vi "CMN_TrimStringWhitespace.vi"(9 "Both Ends?(T)":bool=TRUE, 10 "string":string) -> (3 "trimmed string":string)   [LabVIEW 2016]
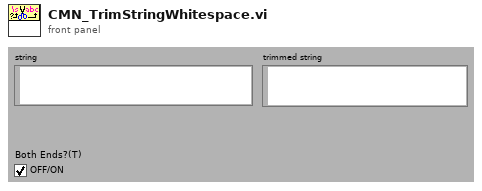
[diagram p1: front panel]
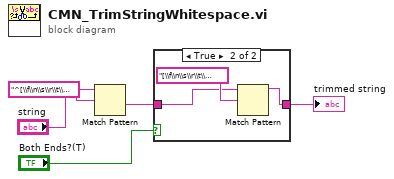
[diagram p0: block diagram]
diagram:
  n1 = Match Pattern(string="string", regular expression="^[\\f\\n\\s\\r\\t\\00]*") -> (after substring=w2:string)  [unwired: 4 out]
  n2 = case shown="True" "Both Ends?(T)" {
    tunnel: w2 -> [w6 w8]
    tunnel: [w6 w7] -> w1
    frame False {
    }
    frame True {
      n3 = Match Pattern(string=w8, regular expression="[\\f\\n\\s\\r\\t\\00]*$") -> (before substring=w7:string)  [unwired: 4 out]
    }
  }
  "trimmed string" <- w1
